vi "limit_deadband.vi"(11 "Val":dbl) -> (3 "Val Out":dbl)   [LabVIEW 2011]
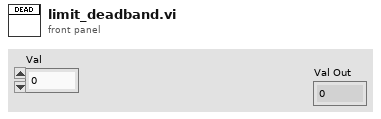
[diagram p1: front panel]
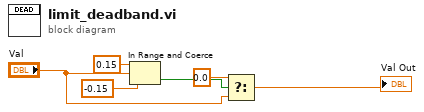
[diagram p0: block diagram]
diagram:
  n1 = In Range and Coerce(upper limit=0.15, x="Val", lower limit=-0.15) -> (In Range?=w4:bool)  [unwired: 1 out]
  n2 = Select(t=0.0, s=w4, f="Val") -> (s? t:f=→"Val Out":dbl)
